vi "02_test.vi"() -> ()   [LabVIEW 2018]
panel:
  out "字符串":string
  out "组合框":string(combo)
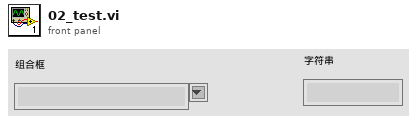
[diagram p1: front panel]
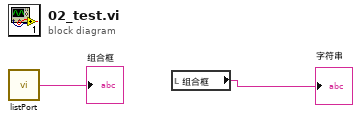
[diagram p0: block diagram]
diagram:
  n1 = call "listPort.vi"() -> ("Combo Box"=→"组合框":string)
  n2 = local read "组合框"() -> (→"字符串":string)
